vi "HELICAL.VI"(0 "Proximal\nRotation Matrix":ext[][](array[numeric]) format="%.2f", 1 "Distal Rotation Matrix":ext[][](array[numeric]) format="%.2f") -> (2 "Vector":ext[](array[numeric]) format="%.2f", 3 "Theta":dbl format="%.2f", 4 "ResolvedToProximal":dbl[](array[numeric]) format="%.2f")   [LabVIEW 2010]
uses:
  <vilib>/Analysis/baseanly.llb/Real A x B.vi
  <vilib>/Analysis/baseanly.llb/Unit Vector (DBL).vi
  <vilib>/Analysis/NI_AALBase.lvlib
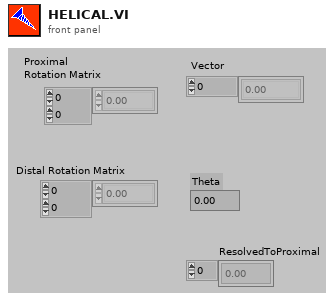
[diagram p1: front panel]
types:
  T1 = typedef "NI_Matrix.lvlib/RealMatrix.ctl" = dbl[][]
  T2 = cluster{"A x B[0]":dbl, "A x B[1]":dbl, "A x B[2]":dbl}
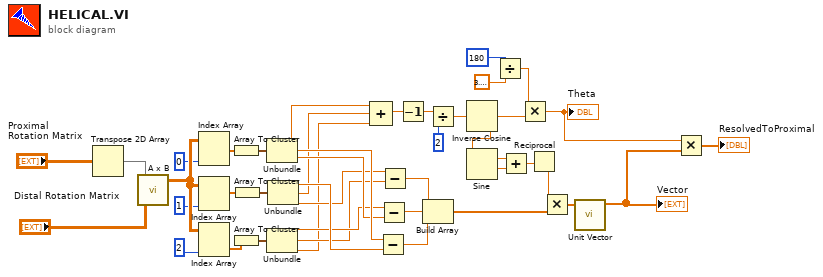
[diagram p0: block diagram]
diagram:
  n1 = Transpose 2D Array(2D array="Proximal\nRotation Matrix") -> (transposed array=w24:ext[][])
  n2 = call-poly <vilib>:"A x B.vi"("B"="Distal Rotation Matrix", "A"=w24) -> ("A x B"=w25:T1)  [unwired: 1 out]
  n3 = Index Array(array=w25, index (col)=0) -> (element=w19:dbl[])  [unwired: 1 in]
  n4 = Index Array(array=w25, index (col)=1) -> (element=w14:dbl[])  [unwired: 1 in]
  n5 = Index Array(array=w25, index (col)=2) -> (element=w9:dbl[])  [unwired: 1 in]
  n6 = Array To Cluster(array=w19) -> (cluster=w20:T2)
  n7 = Array To Cluster(array=w9) -> (cluster=w10:T2)
  n8 = Array To Cluster(array=w14) -> (cluster=w15:T2)
  n9 = Unbundle(w20) -> ("A x B[0]"=w18:dbl, "A x B[1]"=w17:dbl, "A x B[2]"=w16:dbl)
  n10 = Unbundle(w10) -> ("A x B[0]"=w8:dbl, "A x B[1]"=w7:dbl, "A x B[2]"=w6:dbl)
  n11 = Unbundle(w15) -> ("A x B[0]"=w13:dbl, "A x B[1]"=w12:dbl, "A x B[2]"=w11:dbl)
  n12 = Compound Arithmetic op=ADD(w18, w12, w6) -> (w39:dbl)
  n13 = Subtract(x=w17, y=w13) -> (x-y=w30:dbl)
  n14 = Subtract(x=w8, y=w16) -> (x-y=w31:dbl)
  n15 = Subtract(x=w11, y=w7) -> (x-y=w32:dbl)
  n16 = Decrement(x=w39) -> (x-1=w37:dbl)
  n17 = Build Array(w32, w31, w30) -> (w5:dbl[])
  n18 = Divide(x=w37, y=2) -> (x/y=w36:dbl)
  n19 = Inverse Cosine(1:w36) -> (0:w35:dbl)
  n20 = Sine(x=w35) -> (sin(x)=w34:dbl)
  n21 = Divide(x=180, y=3.141592653589793) -> (x/y=w26:dbl)
  n22 = Add(x=w34, y=w34) -> (x+y=w33:dbl)
  n23 = Multiply(x=w26, y=w35) -> (x*y=w3:dbl)
  "Theta" <- w3
  n24 = Reciprocal(x=w33) -> (1/x=w29:dbl)
  n25 = Multiply(x=w29, y=w5) -> (x*y=w4:dbl[])
  n26 = call-poly <vilib>:"Unit Vector.vi"("Input Vector"=w4) -> ("Unit Vector"=w2:dbl[])  [unwired: 8 in, 2 out]
  "Vector" <- w2
  n27 = Multiply(x=w3, y=w2) -> (x*y=→"ResolvedToProximal":dbl[])
